vi "T-periodic Power Exponential Function Normalization.vi"(8 "Error In":errorcluster, 9 "L":i32 caption="Order L", 10 "T":dbl caption="Period T", 11 "tau":dbl caption="Lifetime tau") -> (0 "Error Out":errorcluster, 3 "N(L,tau,T)":dbl)   [LabVIEW 2021, in "Math.lvlib"]
uses:
  <vilib>/gmath/SpecialFunctions.llb/Incomplete Gamma Function.vi
  Math.lvlib
  <vilib>/gmath/NI_Gmath.lvlib
  Time/Time.lvlib
panel:
  out "Time (s)":dbl
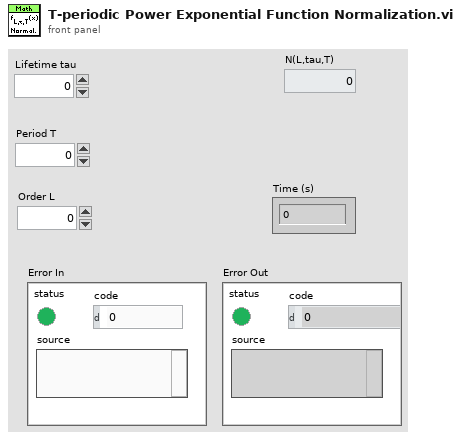
[diagram p1: front panel]
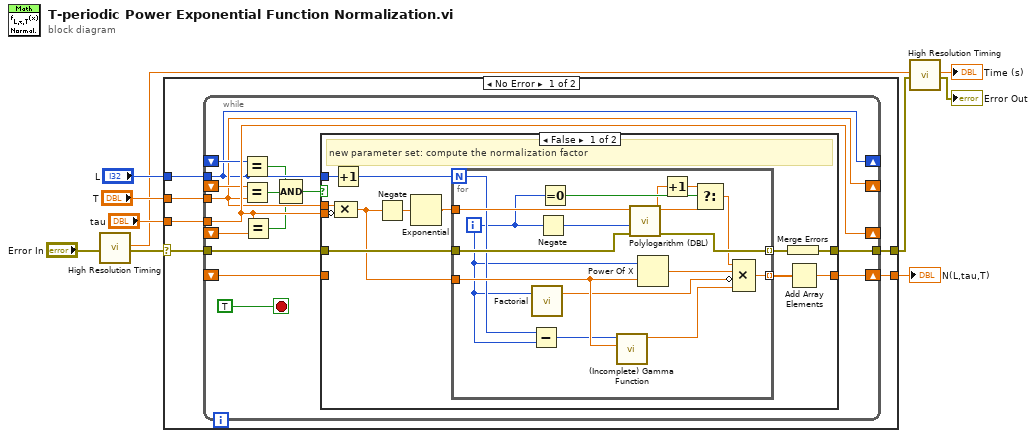
[diagram p0: block diagram]
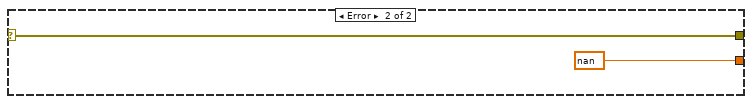
[diagram p3: hidden frame]
diagram:
  n1 = call "High Resolution Timing.vi"("Error In"="Error In") -> ("elapsed (relative) seconds"=w2:dbl, "Error Out"=w4:errorcluster)  [unwired: 16 in, 1 out]
  n2 = case shown="No Error" w4 {
    selector: w4 -> [w15 w63]
    tunnel: "tau" -> [w13 _]
    tunnel: "L" -> [w16 _]
    tunnel: "T" -> [w12 _]
    tunnel: [w14 w63] -> w6
    tunnel: [w11 nan] -> w5
    frame No Error {
      n3 = while {
        tunnel: w16 -> [w22]
        tunnel: w15 -> [w31]
        tunnel: [w30] -> w14
        tunnel: w13 -> [w26]
        tunnel: w12 -> [w23]
        shift-right: [w22] -> _
        shift-left: _ -> [w24]
        shift-right: [w23] -> _
        shift-left: _ -> [w25]
        shift-right: [w26] -> _
        shift-left: _ -> [w27]
        shift-right: [w29] -> w11
        shift-left: _ -> [w17]
        stop <- TRUE stop-if-true
        n4 = Equal?(x=w24, y=w22) -> (x = y?=w20:bool)
        n5 = Equal?(x=w25, y=w23) -> (x = y?=w21:bool)
        n6 = Equal?(x=w26, y=w27) -> (x = y?=w19:bool)
        n7 = Compound Arithmetic op=AND(w20, w21, w19) -> (w18:bool)
        n8 = case shown="False" w18 {
          tunnel: w31 -> [w42 w60]
          tunnel: [w40 w60] -> w30
          tunnel: [w35 w61] -> w29
          tunnel: w26 -> [w34 _]
          tunnel: w23 -> [w33 _]
          tunnel: w22 -> [w32 _]
          tunnel: w17 -> [_ w61]
          frame False {
            # "new parameter set: compute the normalization factor"
            n9 = Increment(x=w32) -> (x+1=w43:i32)
            n10 = Compound Arithmetic op=MULTIPLY(w33, invert w34) -> (w39:dbl)
            n11 = Negate(x=w39) -> (-x=w38:dbl)
            n12 = Exponential(1:w38) -> (0:w37:dbl)
            n13 = for {
              N: w43 -> [w50]
              tunnel: [w54] -> w41 mode=indexing
              tunnel: w42 -> [w55]
              tunnel: w39 -> [w58]
              tunnel: w37 -> [w56]
              tunnel: [w53] -> w36 mode=indexing
              i -> [w48]
              n14 = Subtract(x=w50, y=w48) -> (x-y=w49:i32)
              n15 = call <vilib>:"Factorial.vi"("n"=w48) -> ("n!"=w52:dbl)  [unwired: 2 in]
              n16 = Negate(x=w48) -> (-x=w57:i32)
              n17 = Equal To 0?(x=w48) -> (x = 0?=w47:bool)
              n18 = call-poly <vilib>:"(Incomplete) Gamma Function.vi"("a"=w58, "x"=w49) -> ("g(x, a)"=w51:dbl)  [unwired: 9 in]
              n19 = call "Polylogarithm (DBL).vi"("Error In"=w55, "n"=w57, "z"=w56) -> ("Error Out"=w54:errorcluster, "Li_n(z)"=w46:dbl)  [unwired: 5 in, 2 out]
              n20 = Power Of X(1:w58, 2:w48) -> (0:w59:dbl)
              n21 = Increment(x=w46) -> (x+1=w45:dbl)
              n22 = Select(t=w45, s=w47, f=w46) -> (s? t:f=w44:dbl)
              n23 = Compound Arithmetic op=MULTIPLY(w44, w59, invert w52, w51) -> (w53:dbl)
            }
            n24 = Merge Errors(w41) -> (w40:errorcluster)
            n25 = Add Array Elements(numeric array=w36) -> (sum=w35:dbl)
          }
          frame True {
            # "No need to recompute the normalization factor again"
          }
        }
      }
    }
    frame Error {
    }
  }
  "N(L,tau,T)" <- w5
  n26 = call "High Resolution Timing.vi"("relative seconds (NaN)"=w2, "Error In"=w6) -> ("elapsed (relative) seconds"=→"Time (s)":dbl, "Error Out"=→"Error Out":errorcluster)  [unwired: 15 in, 1 out]
